vi "us open.vi"(8 "error in":errorcluster) -> (0 "error out":errorcluster, 3 "output cluster":refnum<class "US sensor.lvclass">)   [LabVIEW 2019]
uses:
  FPGA_subVIs/low level/us sensor/US sensor.lvclass
  FPGA_subVIs/low level/us sensor/us select.ctl
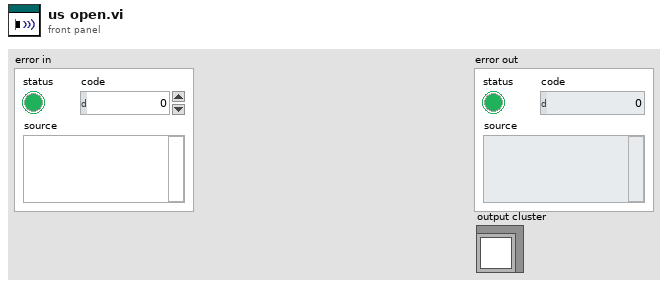
[diagram p1: front panel]
types:
  T1 = typedef "my FPGA lib.lvlib/US sensor.lvclass/us select.ctl" = enum16{"US.1", "US.2", "US.3", "US.4"}
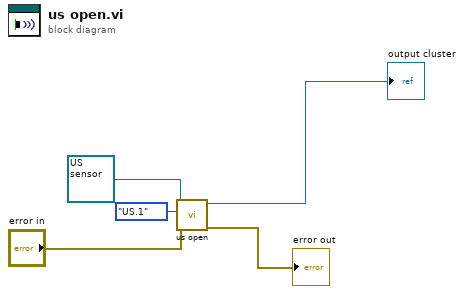
[diagram p0: block diagram]
diagram:
  n1 = call "us open.vi"("error in"="error in", "Enum"=us_select."US.1", "my FPGA lib.lvlib:US sensor.lvclass"=refnum<class "US sensor.lvclass"> refnum) -> ("error out"=→"error out":errorcluster, "output cluster"=→"output cluster":refnum<class "US sensor.lvclass">)  [unwired: 7 in]
